vi "Configuration File Handler.vi"(8 "error in":errorcluster, 10 "selected configuration file":path, 11 "configuration file page data":T1 {"custom device ref" format="%.0x"}) -> (0 "error out":errorcluster, 3 "configuration file page data out":T1 {"custom device ref" format="%.0x"})   [LabVIEW 2020, in "AIM ARINC 664 System Explorer.lvlib" / "Implementation.lvlib"]
uses:
  Implementation.lvlib
  Types/Configuration File Page Data.ctl
  Types/Path Control.ctl
  Types/Browse Button.ctl
  <vilib>/NI VeriStand/Custom Device API/Custom Device Item Ref.ctl
  Scripting/AIM ARINC 664 Scripting.lvlib
  Import/AIM ARINC 664 Import.lvlib
  <vilib>/NI VeriStand/Custom Device API/Custom Device API.lvlib
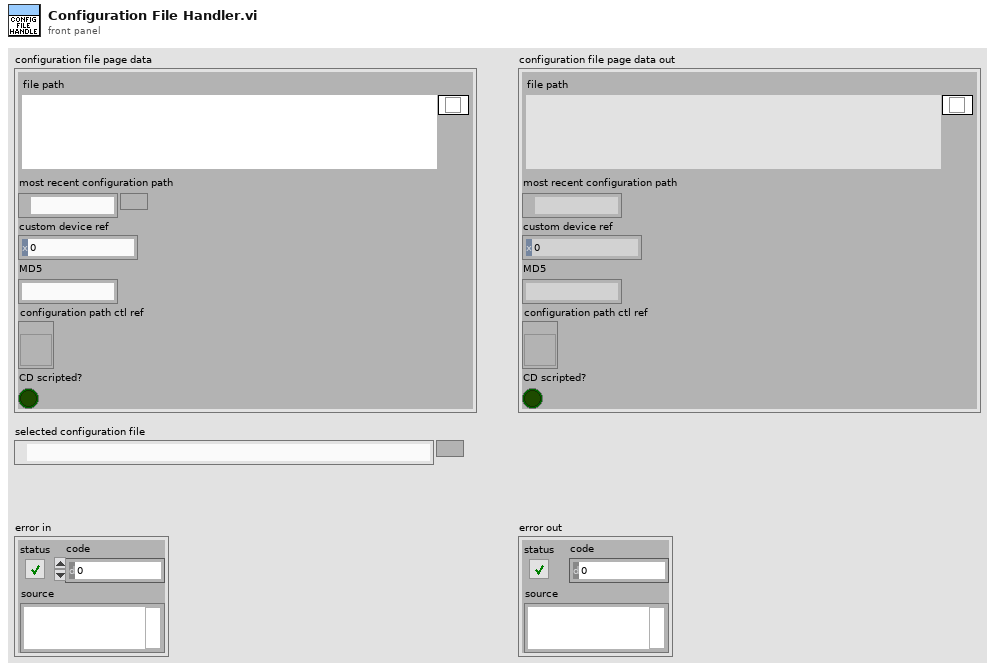
[diagram p1: front panel]
types:
  T1 = typedef "AIM ARINC 664 System Explorer.lvlib/Implementation.lvlib/Configuration File Page Data.ctl" = cluster{"Parameters":T2, "most recent configuration path":path, "custom device ref":T4, "MD5":string, "configuration path ctl ref":refnum<vi>, "CD scripted?":bool}
  T2 = typedef "AIM ARINC 664 System Explorer.lvlib/Implementation.lvlib/Path Control.ctl" = cluster{"file path":path, "Browse":T3}
  T3 = typedef "AIM ARINC 664 System Explorer.lvlib/Implementation.lvlib/Browse Button.ctl" = bool
  T4 = typedef "Custom Device API.lvlib/Custom Device Item Ref.ctl" = u64
  T5 = typedef "Port Session Configuration.ctl" = cluster{"boardId":u32, "session_tx_generic":T6[], "session_rx_monitor":T7[]}
  T6 = typedef "session_tx_generic.ctl" = cluster{"portId":u32, "QueueSizeIn":u32}
  T7 = typedef "session_rx_monitor.ctl" = cluster{"portId":u32, "DefaultCronoMode":u32, "GlbMonBufferSizeIn":u32, "CaptureMode":u32, "MaxFileSize MB (1)":u32, "Strobe":u32, "TriggerPosition":u32}
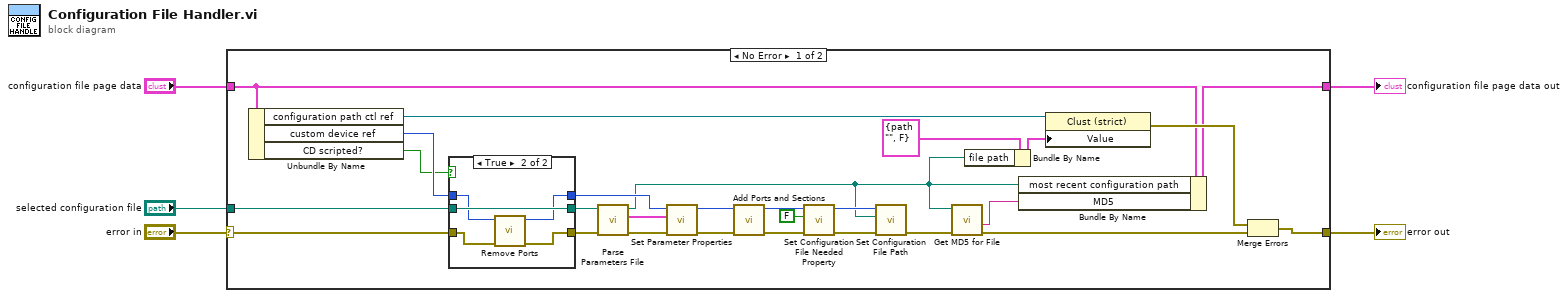
[diagram p0: block diagram]
diagram:
  n1 = case shown="No Error" "error in" {
    selector: "error in" -> [w19 w41]
    tunnel: "configuration file page data" -> [w31 w42]
    tunnel: "selected configuration file" -> [w20 _]
    tunnel: [w14 w42] -> w2
    tunnel: [w30 w41] -> w1
    frame No Error {
      n2 = Unbundle By Name(w31) -> ("configuration path ctl ref"=w29:refnum<vi>, "custom device ref"=w16:T4, "CD scripted?"=w11:bool)
      n3 = case shown="True" w11 {
        tunnel: w20 -> [w34 w40]
        tunnel: w19 -> [w35 w39]
        tunnel: [w35 w38] -> w18
        tunnel: [w34 w40] -> w17
        tunnel: w16 -> [w33 w37]
        tunnel: [w33 w36] -> w15
        frame False {
        }
        frame True {
          n4 = call "Remove Ports.vi"("error in"=w39, "Custom device Ref"=w37) -> ("error out"=w38:errorcluster, "Custom device Ref out"=w36:T4)  [unwired: 8 in]
        }
      }
      n5 = call "Parse Parameters File.vi"("error in"=w18, "path to XML document"=w17) -> ("error out"=w23:errorcluster, "port sessions"=w28:T5, "path to XML document out"=w6:path)  [unwired: 7 in]
      n6 = call "Set Parameter Properties.vi"("custom device ref in"=w15, "port sessions"=w28, "error in"=w23) -> ("custom device ref out"=w21:T4, "error out"=w27:errorcluster)  [unwired: 6 in]
      n7 = call "Add Ports and Sections.vi"("error in"=w27, "custom device ref"=w21) -> ("error out"=w22:errorcluster, "custom device ref out"=w13:T4)  [unwired: 8 in]
      n8 = call "Set Configuration File Needed Property.vi"("error in"=w22, "needed?"=FALSE, "custom device ref in"=w13) -> ("error out"=w10:errorcluster, "custom device ref out"=w7:T4)  [unwired: 7 in]
      n9 = call "Set Configuration File Path.vi"("error in"=w10, "configuration file path"=w6, "custom device ref in"=w7) -> ("error out"=w8:errorcluster)  [unwired: 7 in, 1 out]
      n10 = call "Get MD5 for File.vi"("error in"=w8, "Path"=w6) -> ("error out"=w9:errorcluster, "MD5"=w26:string)  [unwired: 8 in]
      n11 = Bundle By Name(cluster=T2 {"file path"=path "", "Browse"=FALSE} ("Path"), "file path"=w6) -> (w24:T2)
      n12 = Bundle By Name(cluster=w31, "most recent configuration path"=w6, "MD5"=w26) -> (w14:T1)
      n13 = property class="Clust (strict)"(reference=w29, "Value"=w24) -> (error out=w32:errorcluster)  [unwired: 1 in, 1 out]
      n14 = Merge Errors(w32, w9) -> (w30:errorcluster)
    }
    frame Error {
    }
  }
  "configuration file page data out" <- w2
  "error out" <- w1
